vi "SendMessage.vi"(0 "reference in":refnum<class "Mediator.lvclass">, 2 "Sender":string, 4 "Receiver":string, 5 "error in (no error)":errorcluster, 8 "Message":string) -> (14 "reference out":refnum<class "Mediator.lvclass">, 19 "error out":errorcluster)   [LabVIEW 2013, in "Mediator.lvclass"]
uses:
  Mediator.lvclass
  Colleague_class/Colleague.lvclass
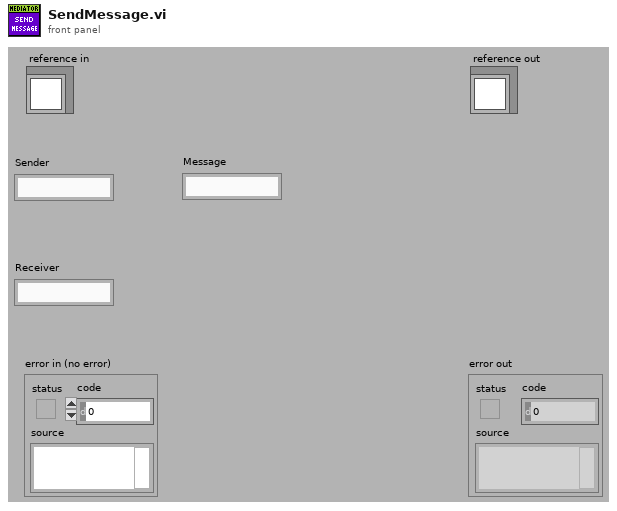
[diagram p1: front panel]
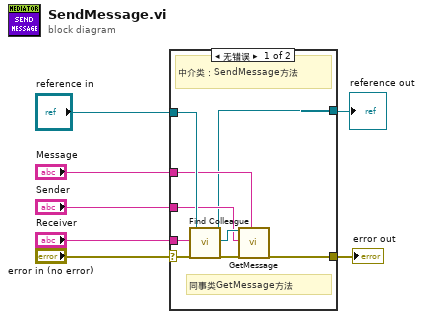
[diagram p0: block diagram]
diagram:
  n1 = case shown="无错误" "error in (no error)" {
    selector: "error in (no error)" -> [w11 w18]
    tunnel: [w9 w18] -> w6
    tunnel: [w8 w17] -> w4
    tunnel: "reference in" -> [w16 w17]
    tunnel: "Receiver" -> [w15 _]
    tunnel: "Message" -> [w14 _]
    tunnel: "Sender" -> [w12 _]
    frame No Error {
      # "同事类GetMessage方法"
      # "中介类：SendMessage方法"
      n2 = call "Find Colleague.vi"("reference in"=w16, "Name"=w15, "error in (no error)"=w11) -> ("reference out"=w8:refnum<class "Mediator.lvclass">, "Colleague.lvclass"=w13:refnum<class "Colleague.lvclass">, "error out"=w10:errorcluster)  [unwired: 14 in]
      n3 = call-dynamic "GetMessage.vi"("reference in"=w13, "Sender"=w12, "error in (no error)"=w10, "Message"=w14) -> ("error out"=w9:errorcluster)  [unwired: 14 in, 1 out]
    }
    frame Error {
    }
  }
  "error out" <- w6
  "reference out" <- w4
